vi "Accelerator_DAQ_Small.vi"() -> ()   [LabVIEW 2013]
doc: "Acquire Accelerator Data"
uses:
  <instrlib>/niScope/Controls/niScope vertical coupling.ctl
  <instrlib>/niScope/Controls/niScope trigger slope.ctl
  <instrlib>/niScope/Controls/niScope trigger coupling.ctl
  <instrlib>/niScope/Controls/niScope trigger source.ctl
  Accelerator Measurement/Array_Defctl.ctl
  <vilib>/Utility/error.llb/DialogType.ctl
  <vilib>/Utility/miscctls.llb/LVPointTypeDef.ctl
  Public API/Dust_Event.ctl
  Public API/Signal.ctl
  Private/Role ID.ctl
  Private/Hardware ID.ctl
  Private/Estimate_source.ctl
  Functional Global Variables/Action Items.ctl
  <vilib>/Analysis/baseanly.llb/Mean (DBL).vi
  Private/PSU updated.vi
  <vilib>/addons/database/Connection.llb/Conn Execute.vi
  <vilib>/addons/database/Recordset.llb/Rec Fetch Recordset Data (R).vi
  <vilib>/addons/database/Recordset.llb/Rec Destroy - Connection.vi
  <instrlib>/niScope/Configure/Trigger/niScope Configure Trigger Edge.vi
  <instrlib>/niScope/Acquire/Fetch/niScope Multi Fetch Cluster.vi
  <vilib>/addons/database/_DB Variant To Data/Database Variant To Data.xnode
  <vilib>/Analysis/NI_AALBase.lvlib
  <vilib>/addons/database/NI_Database_API.lvlib
panel:
  out "Big Accelerator?":bool
  out "Array 2":T1=["Dev1", "Dev2"]
  out "error out 5":errorcluster
  in  "Trigger":enum32{"Edge"}(tab)
  in  "Trigger Source Edge 2":T2="2" caption="Source"
  in  "Trigger Source Edge":T2="0" caption="Source"
  in  "Coupling":T3=1 items=["AC"=0, "DC"=1, "HF Reject"=3, "LF Reject"=4, "AC Plus HF Reject"=1001]
  in  "Slope":T4 caption="Trigger Slope"
  in  "Level":dbl=1.0 caption="Trigger Level" step=0.001 format="%.3f"
  in  "Delay":dbl caption="Trigger Delay" format="%.4p"
  in  "Reference Position (%)":dbl=40.0 caption="Ref Position" format="%.1f"
  in  "Bandwidth":dbl=-1.0 format="%.2f"
  in  "Vertical Coupling":T5=1 items=["AC", "DC", "Ground"]
  in  "Probe Attenuation":dbl=1.0 format="%.1f"
  in  "Vertical Offset":dbl format="%.4f"
  in  "Vertical Range":dbl=5.0 caption="Vertical Range (V)" format="%.2f"
  out "Actual Sample Rate":dbl=10000000.0 format="%.0p"
  in  "Min Record Length":i32=100000 caption="Min. Record Length"
  in  "Min Sample Rate":dbl=80000000.0 caption="Min. Sample Rate" step=1000000.0 format="%.2p"
  out "Actual Record Length":i32=100000
  out "Mass":dbl format="%#_3g"
  in  "Write to Database?":bool=TRUE
  in  "Limit":dbl
  in  "Limit Triggers":bool
  out "Acquisition #":i32
  in  "WFM Tag":string="trace"
  in  "Location":string="G:\\default"
  in  "Write Raw File?":bool
  out "Saving Raw File...":path=path "G:/2012_06_13_verify_timestamp_labview/trace00000"
  out "?":cluster{dbl, dbl}(knob)={0.0549, 2.0} scale=10.0..0.01
  in  "Ideal Time (Cursor)":dbl=2.0 step=0.01 format="%_2f"
  out "Time Between Triggers":dbl
  out "Average Frequency":dbl format="%#_4g"
  out "output cluster":T6
  out "error out 3":errorcluster
  out "# elements in queue":i32
  out "Stop condition":bool=TRUE
  out "created path":path=path "G:/default"
  out "Numeric":i32=92364
  out "error out 2":errorcluster
  out "Calibration":dbl=24700000000000.0
  out "Array":T1=["Dev1", "Dev2"]
  in  "Debug Mode\n(Confusing)":bool
  out "Multi Plot 2":cluster{dbl[], dbl[]}(graph) caption="Multi Plot"
  in  "Acceleration Voltage (MV)":dbl=2.0 format="%_2g"
  out "Charge":dbl format="%#_3g"
  out "Velocity (Est.)":dbl format="%#_6f"
  out "Final Detector (CH3)":waveform(dbl)(graph)={"t0"=timestamp(0 s since 1904-01-01), "dt"=1e-07, "Y"=[]}
  out "Charge Detector/PSU gate (CH2)":waveform(dbl)(graph)={"t0"=timestamp(0 s since 1904-01-01), "dt"=1e-07, "Y"=[]}
  out "Velocity Detectors (CH0 & CH1)":waveform(dbl)[](graph)
  in  "stop":bool=TRUE
  out "error out":errorcluster={"status"=FALSE, "code"=0, "source"="No Error"} {"code" format="%.0x"}
  # "File Parameters"
  # "Error Handling"
  # "Accelerator DAQ"
  # "Trigger"
  # "Channel"
  # "Vertical"
  # "Horizontal"
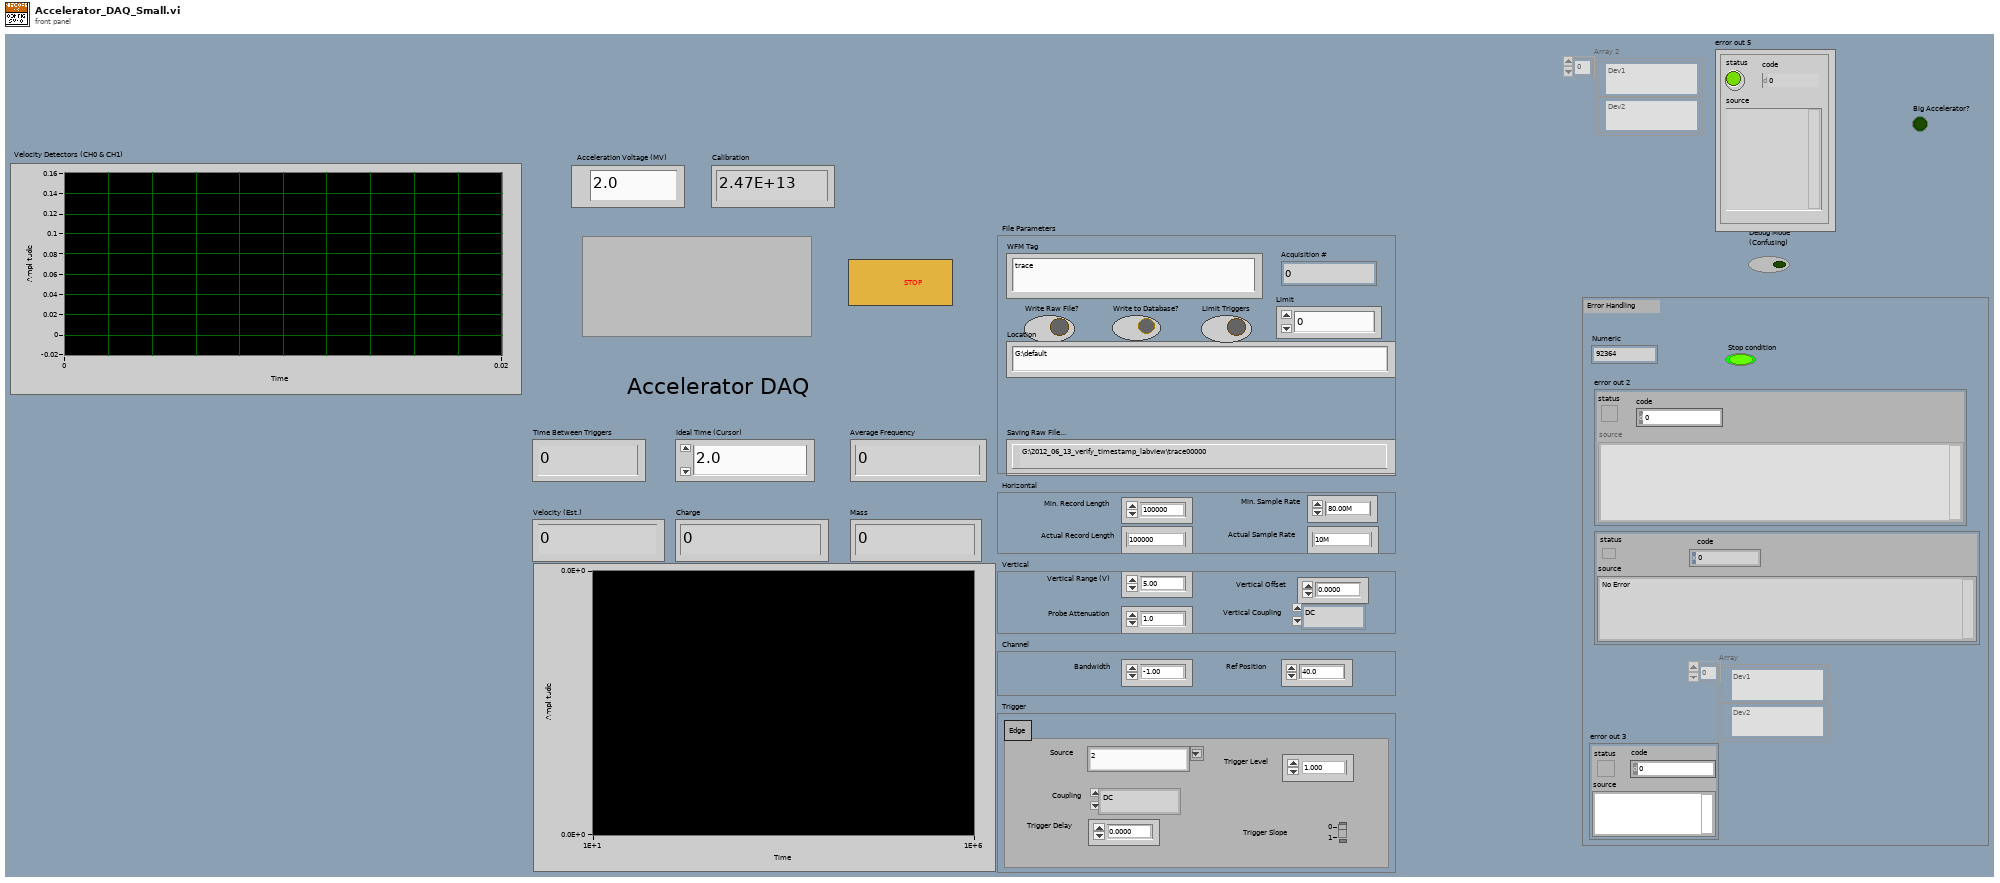
[diagram p1: front panel]
types:
  T1 = typedef "Array_Defctl.ctl" = refnum<k15>[]
  T2 = typedef "niScope trigger source.ctl" = string
  T3 = typedef "niScope trigger coupling.ctl" = u16
  T4 = typedef "niScope trigger slope.ctl" = i32
  T5 = typedef "niScope vertical coupling.ctl" = i32
  T6 = cluster{"File Path Control":path, "Array":waveform(dbl)[]}
  T7 = typedef "LVPointTypeDef.ctl" = cluster{"Horizontal":i16, "Vertical":i16}
  T8 = typedef "DialogType.ctl" = u16
  T9 = typedef "LVAllMonitorsDisplayTypeDef.ctl" = cluster{"Bounds":cluster{"Left":i16, "Top":i16, "Right":i16, "Bottom":i16}, "Depth":i16}[]
  T10 = cluster{"Bounds":cluster{"Left":i16, "Top":i16, "Right":i16, "Bottom":i16}, "Depth":i16}
  T11 = cluster{"Left":i16, "Top":i16, "Right":i16, "Bottom":i16}
  T12 = typedef "NI_Database_API.lvlib/Conn ObjectReference.ctl" = refnum<k1>
  T13 = typedef "NI_Database_API.lvlib/Rec ObjectReference.ctl" = refnum<k1>
  T14 = cluster{"Integer Timestamp":dbl, "Max Velocity":dbl, "Min Velocity":dbl}
  T15 = cluster{"first point time":dbl, "xIncrement":dbl, "Waveforms":dbl[]}[]
  T16 = typedef "Dust_Event.ctl" = cluster{"Time Stamp":timestamp, "Velocity":sgl, "Mass":sgl, "Charge":sgl, "Radius":sgl, "Array":T17[], "Dust Event ID":i64, "Passed_3rd_Detector":bool, "Estimate Source":T20, "Estimate Quality":sgl}
  T17 = typedef "Signal.ctl" = cluster{"Signal ID":i64, "Time Stamp":timestamp, "Dust Event ID":i64, "Role ID":T18, "Data":sgl[], "Signal Length":i32, "dt":sgl, "Offset":dbl, "Hardware ID":T19}
  T18 = typedef "Role ID.ctl" = enum16{"First_Detector", "Second_Detector", "Third_Detector", "LeCroy_CH1", "LeCroy_CH2", "LeCroy_CH3", "LeCroy_CH4", "PSU"}
  T19 = typedef "Hardware ID.ctl" = enum16{"Unknown", "CSA 1", "CSA 2", "CSA 3", "CSA 4", "CSA 5", "CSA 6"}
  T20 = typedef "Estimate_source.ctl" = i8
  T21 = typedef "Action Items.ctl" = enum16{"Initialize", "Get", "Set"}
  T22 = cluster{"relativeInitialX":dbl, "xIncrement":dbl, "wfm":dbl[]}[]
  T23 = cluster{"first point time":dbl, "xIncrement":dbl, "Waveforms":dbl[]}
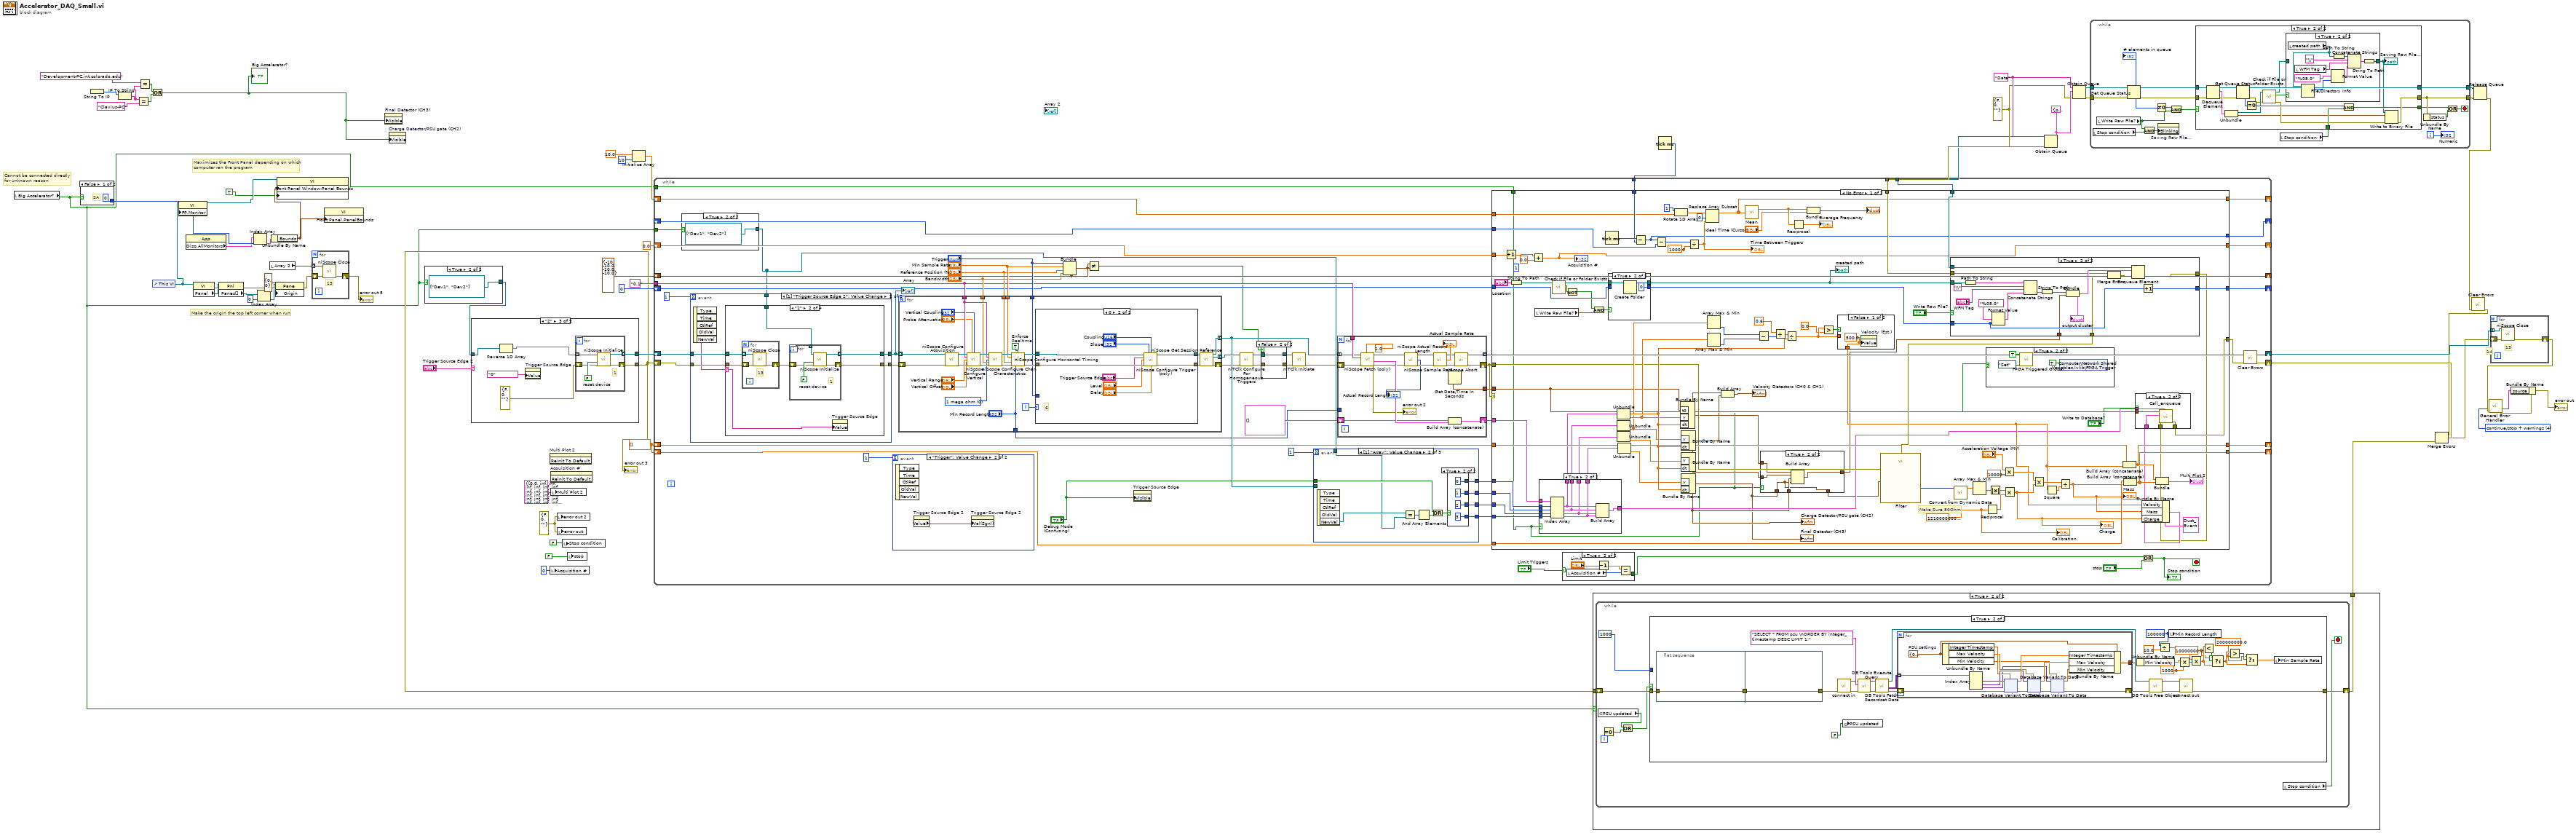
[diagram p0: block diagram]
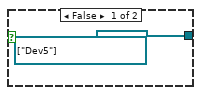
[diagram p2: hidden frame]
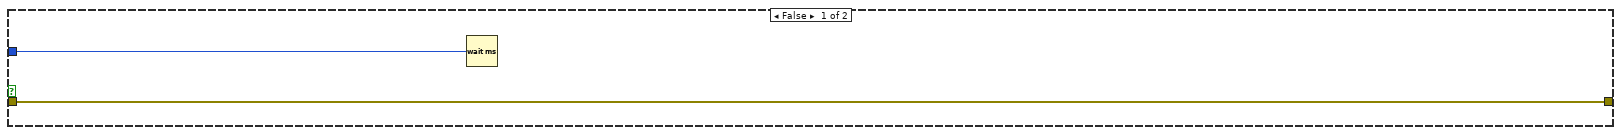
[diagram p4: hidden frame]
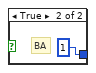
[diagram p5: hidden frame]
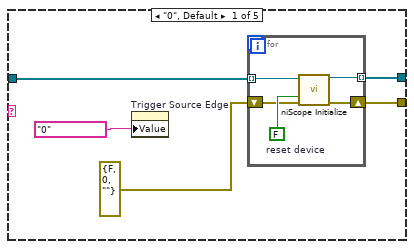
[diagram p6: hidden frame]
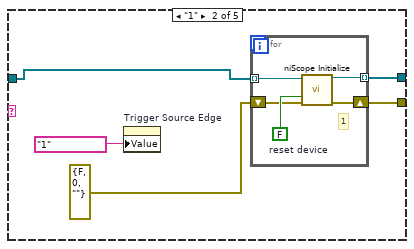
[diagram p7: hidden frame]
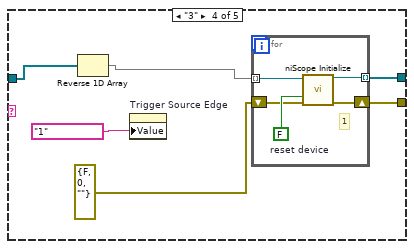
[diagram p8: hidden frame]
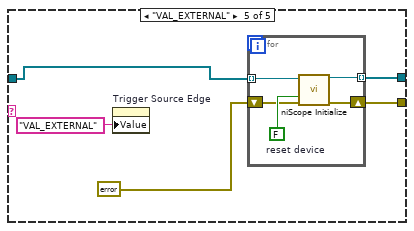
[diagram p9: hidden frame]
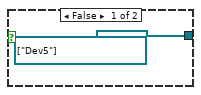
[diagram p10: hidden frame]
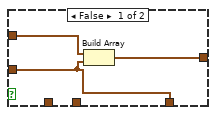
[diagram p11: hidden frame]
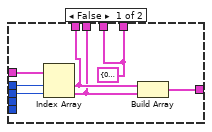
[diagram p12: hidden frame]
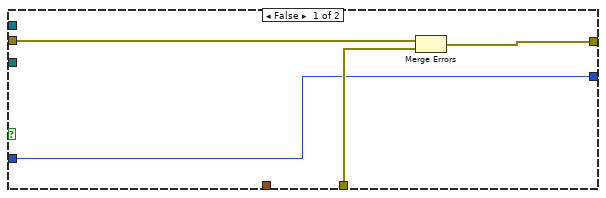
[diagram p16: hidden frame]
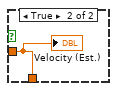
[diagram p17: hidden frame]
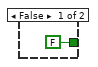
[diagram p19: hidden frame]
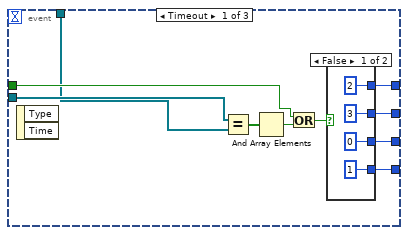
[diagram p20: hidden frame]
diagram:
  w31 = dbl[] []
  w38 = errorcluster {"status"=FALSE, "code"=0, "source"=""} ("error out")
  w42 = errorcluster {"status"=FALSE, "code"=0, "source"=""} ("error out")
  w43 = cluster{path, waveform(sgl)[]} {path "", []} ("output cluster")
  w44 = "Data" ("name (unnamed)")
  w36 = T8 4 items=["no dialog", "OK message", "continue or stop message", "OK message + warnings", "continue/stop + warnings"] ("type of dialog (OK msg:1)")
  # "Cannot be connected directly\nfor unknown reason"
  # "Maximizes the Front Panel depending on which\ncomputer ran the program"
  # "Make the origin the top left corner when run"
  # "14"
  n1 = local read "Big Accelerator?"() -> (w1:bool)
  n2 = case shown="False" w1 {
    tunnel: [0 1] -> w10
    frame False {
      # "SA"
    }
    frame True {
      # "BA"
    }
  }
  n3 = String To IP() -> (0:w16:u32)  [unwired: 1 in]
  n4 = IP To String(2:w16) -> (0:w13:string)  [unwired: 1 in]
  n5 = Equal?(x=w13, y="Clavius-PC") -> (x = y?=w5:bool)
  n6 = Equal?(x="Development-PC.int.colorado.edu", y=w13) -> (x = y?=w4:bool)
  n7 = Or(x=w4, y=w5) -> (x .or. y?=w3:bool)
  "Big Accelerator?" <- w3
  n8 = control-ref of="This VI"() -> (w11:refnum<vi>)
  n9 = property class="VI"(reference=w11, "FP.Monitor"=w10) -> (reference out=w7:refnum<vi>)  [unwired: 1 in, 1 out]
  n10 = property class="App"() -> ("Disp.AllMonitors"=w9:T9)  [unwired: 2 in, 2 out]
  n11 = property class="VI"(reference=w11) -> (error out=w23:errorcluster, "Panel"=w12:refnum<vi>)  [unwired: 1 in, 1 out]
  n12 = property class="Pnl"(reference=w12, error in=w23) -> (error out=w22:errorcluster, "Panes[]"=w21:refnum<vi>[])  [unwired: 1 out]
  n13 = Index Array(array=w9, index=w10) -> (element=w8:T10)
  n14 = Index Array(array=w21, index=0) -> (element=w19:refnum<vi>)
  n15 = local read "Array 2"() -> (w25:T1)
  n16 = Unbundle By Name(w8) -> ("Bounds"=w6:T11)
  n17 = property class="Pane"(reference=w19, error in=w22, "Origin"=T7 {"Horizontal"=0, "Vertical"=0}) -> (error out=w17:errorcluster)  [unwired: 1 out]
  n18 = property class="VI"(reference=w7, "Front Panel Window:Panel Bounds"=w6, "Front Panel Window:Size to Screen (Deprecated)"=TRUE) -> ()  [unwired: 1 in, 2 out]
  n19 = for {
    tunnel: w25 -> [w66] mode=indexing
    shift-right: [w68] -> w24
    shift-left: w17 -> [w67]
    # "13"
    n20 = call <instrlib>:"niScope Close.vi"("instrument handle"=w66, "error in"=w67) -> ("error out"=w68:errorcluster)  [unwired: 13 in]
  }
  "error out 5" <- w24
  n21 = property class="VI"("Front Panel.PanelBounds"=w6) -> ()  [unwired: 2 in, 2 out]
  n22 = property on="Final Detector (CH3)" class="WFGraph (strict)"("Visible"=w3) -> ()  [unwired: 2 in, 2 out]
  n23 = property on="Charge Detector/PSU gate (CH2)" class="WFGraph (strict)"("Visible"=w3) -> ()  [unwired: 2 in, 2 out]
  n24 = case shown="True" w1 {
    tunnel: [refnum<k15>[] ["Dev5"] ("Resources") refnum<k15>[] ["Dev1", "Dev2"] ("Resources")] -> w26
    frame False {
    }
    frame True {
    }
  }
  n25 = case shown="\"2\"" "Trigger Source Edge 2" {
    tunnel: [w75 w84 w95 w106 w117] -> w62
    tunnel: [w74 w83 w94 w105 w116] -> w29
    tunnel: w26 -> [w71 w81 w92 w103 w113]
    frame "0", Default {
      n26 = property on="Trigger Source Edge" class="CmbBox (strict)"("Value"=T2 "0" ("Trigger Source Edge")) -> ()  [unwired: 2 in, 2 out]
      n27 = for {
        tunnel: w71 -> [w79] mode=indexing
        tunnel: [w77] -> w75 mode=indexing
        shift-right: [w76] -> w74
        shift-left: errorcluster {"status"=FALSE, "code"=0, "source"=""} ("error out") -> [w78]
        w80 = FALSE  # reset device
        n28 = call <instrlib>:"niScope Initialize.vi"("resource name"=w79, "reset device"=w80, "error in"=w78) -> ("instrument handle"=w77:refnum<k15>, "error out"=w76:errorcluster)  [unwired: 11 in]
      }
    }
    frame "1" {
      n29 = property on="Trigger Source Edge" class="CmbBox (strict)"("Value"=T2 "1" ("Trigger Source Edge")) -> ()  [unwired: 2 in, 2 out]
      n30 = for {
        tunnel: w81 -> [w89] mode=indexing
        tunnel: [w87] -> w84 mode=indexing
        shift-right: [w86] -> w83
        shift-left: errorcluster {"status"=FALSE, "code"=0, "source"=""} ("error out") -> [w88]
        w90 = FALSE  # reset device
        # "1"
        n31 = call <instrlib>:"niScope Initialize.vi"("resource name"=w89, "reset device"=w90, "error in"=w88) -> ("instrument handle"=w87:refnum<k15>, "error out"=w86:errorcluster)  [unwired: 11 in]
      }
    }
    frame "2" {
      n32 = Reverse 1D Array(array=w92) -> (reversed array=w91:refnum<k15>[])
      n33 = property on="Trigger Source Edge" class="CmbBox (strict)"("Value"=T2 "0" ("Trigger Source Edge")) -> ()  [unwired: 2 in, 2 out]
      n34 = for {
        tunnel: w91 -> [w100] mode=indexing
        tunnel: [w98] -> w95 mode=indexing
        shift-right: [w97] -> w94
        shift-left: errorcluster {"status"=FALSE, "code"=0, "source"=""} ("error out") -> [w99]
        w101 = FALSE  # reset device
        # "1"
        n35 = call <instrlib>:"niScope Initialize.vi"("resource name"=w100, "reset device"=w101, "error in"=w99) -> ("instrument handle"=w98:refnum<k15>, "error out"=w97:errorcluster)  [unwired: 11 in]
      }
    }
    frame "3" {
      n36 = Reverse 1D Array(array=w103) -> (reversed array=w102:refnum<k15>[])
      n37 = property on="Trigger Source Edge" class="CmbBox (strict)"("Value"=T2 "1" ("Trigger Source Edge")) -> ()  [unwired: 2 in, 2 out]
      n38 = for {
        tunnel: w102 -> [w111] mode=indexing
        tunnel: [w109] -> w106 mode=indexing
        shift-right: [w108] -> w105
        shift-left: errorcluster {"status"=FALSE, "code"=0, "source"=""} ("error out") -> [w110]
        w112 = FALSE  # reset device
        # "1"
        n39 = call <instrlib>:"niScope Initialize.vi"("resource name"=w111, "reset device"=w112, "error in"=w110) -> ("instrument handle"=w109:refnum<k15>, "error out"=w108:errorcluster)  [unwired: 11 in]
      }
    }
    frame "VAL_EXTERNAL" {
      n40 = property on="Trigger Source Edge" class="CmbBox (strict)"("Value"=T2 "VAL_EXTERNAL" ("Trigger Source Edge")) -> ()  [unwired: 2 in, 2 out]
      n41 = for {
        tunnel: w113 -> [w121] mode=indexing
        tunnel: [w119] -> w117 mode=indexing
        shift-right: [w118] -> w116
        shift-left: errorcluster {"status"=FALSE, "code"=0, "source"=""} ("error out") -> [w120]
        w122 = FALSE  # reset device
        n42 = call <instrlib>:"niScope Initialize.vi"("resource name"=w121, "reset device"=w122, "error in"=w120) -> ("instrument handle"=w119:refnum<k15>, "error out"=w118:errorcluster)  [unwired: 11 in]
      }
    }
  }
  "error out 3" <- w29
  n43 = invoke on="Multi Plot 2" class="XYGraph (strict)" method="Reinit To Default"() -> ()  [unwired: 3 in, 3 out]
  n44 = local write "Acquisition #"(0 ("Acquisition #")) -> ()
  n45 = invoke on="Acquisition #" class="DigNum (strict)" method="Reinit To Default"() -> ()  [unwired: 3 in, 3 out]
  n46 = local write "Multi Plot 2"(cluster{dbl[], dbl[]} {[0.0, inf, inf, inf, inf, inf, inf, inf, inf, inf, inf, inf, inf, inf, inf, inf, inf, inf, inf, inf, inf, inf, inf, inf, inf, inf, inf, inf, inf, inf, inf, inf, inf, inf, inf, inf, inf, inf, inf, inf, inf], [0.0, 0.0, 0.0, 0.0, 0.0, 0.0, 0.0, 0.0, 0.0, 0.0, 0.0, 0.0, 0.0, 0.0, 0.0, 0.0, 0.0, 0.0, 0.0, 0.0, 0.0, 0.0, 0.0, 0.0, 0.0, 0.0, 0.0, 0.0, 0.0, 0.0, 0.0, 0.0, 0.0, 0.0, 0.0, 0.0, 0.0, 0.0, 0.0, 0.0, 0.0]} ("Multi Plot 2")) -> ()
  n47 = local write "error out 2"(w38) -> ()
  n48 = local write "error out"(w38) -> ()
  n49 = local write "Stop condition"(FALSE ("x .or. y?")) -> ()
  n50 = local write "stop"(FALSE ("stop")) -> ()
  n51 = Initialize Array(10.0 ("element"), 10 ("dimension size")) -> (w54:dbl[])
  n52 = case shown="True" w1 {
    tunnel: w29 -> [w123 w125]
    tunnel: [w123 w124] -> w28
    frame False {
    }
    frame True {
      n53 = while {
        shift-right: [w132] -> w124
        shift-left: w125 -> [w133]
        i -> [w131]
        stop <- w130 stop-if-true
        n54 = global read "PSU updated.vi" "PSU updated"() -> (w129:bool)
        n55 = Equal To 0?(x=w131) -> (x = 0?=w127:bool)
        n56 = Or(x=w129, y=w127) -> (x .or. y?=w128:bool)
        n57 = case shown="True" w128 {
          tunnel: w133 -> [w134 w164]
          tunnel: [w134 w163] -> w132
          tunnel: 1000 -> [w135 _]
          frame False {
            n58 = Wait (ms)(milliseconds to wait=w135) -> ()  [unwired: 1 out]
          }
          frame True {
            w137 = 200000000.0 ("y")
            w140 = 10000000.0 ("y")
            w147 = 100000 ("Min Record Length")
            n59 = flat-sequence {
              tunnel: [w166] -> w165
              tunnel: w164 -> [w166]
              tunnel: w165 -> [w167]
              tunnel: [w167] -> w150
              frame #0 {
              }
              frame #1 {
              }
            }
            n60 = call "connect in.vi"("error in (no error)"=w150) -> ("error out"=w154:errorcluster, "Database Connection"=w153:T12)  [unwired: 6 in, 1 out]
            n61 = global write "PSU updated.vi" "PSU updated"(FALSE ("PSU updated")) -> ()
            n62 = call-poly <vilib>:"DB Tools Execute Query.vi"("error in (no error)"=w154, "SQL query"="SELECT * FROM psu \nORDER BY integer_timestamp DESC LIMIT 1;", "connection reference"=w153) -> ("error out"=w156:errorcluster, "recordset reference"=w155:T13)  [unwired: 5 in]
            n63 = call-poly <vilib>:"DB Tools Fetch Recordset Data.vi"("error in (no error)"=w156, "recordset reference"=w155) -> ("error out"=w162:errorcluster, "recordset data"=w161:variant[][], "recordset reference out"=w157:T13)  [unwired: 3 in]
            n64 = for {
              tunnel: w161 -> [w183] mode=indexing
              shift-right: [w168] -> w151
              shift-left: w162 -> [w179]
              tunnel: [w178] -> w152
              w173 = T14 {"Integer Timestamp"=0.0, "Max Velocity"=0.0, "Min Velocity"=0.0}  # PSU settings
              n65 = Unbundle By Name(w173) -> ("Integer Timestamp"=w177:dbl, "Max Velocity"=w174:dbl, "Min Velocity"=w171:dbl)
              n66 = Index Array(array=w183) -> (element #1=w182:variant, element #2=w181:variant, element #3=w172:variant)  [unwired: 3 in]
              n67 = xnode "Database Variant To Data"("database variant"=w182, "error in"=w179, "type"=w177) -> ("data"=w176:dbl, "error out"=w180:errorcluster)
              n68 = xnode "Database Variant To Data"("database variant"=w181, "error in"=w180, "type"=w174) -> ("data"=w175:dbl, "error out"=w169:errorcluster)
              n69 = xnode "Database Variant To Data"("database variant"=w172, "error in"=w169, "type"=w171) -> ("data"=w170:dbl, "error out"=w168:errorcluster)
              n70 = Bundle By Name(cluster=w173, "Integer Timestamp"=w176, "Max Velocity"=w175, "Min Velocity"=w170) -> (w178:T14)
            }
            n71 = Unbundle By Name(w152) -> ("Min Velocity"=w146:dbl)
            n72 = call-poly <vilib>:"DB Tools Free Object.vi"("error in (no error)"=w151, "recordset reference"=w157) -> ("error out"=w158:errorcluster, "connection reference"=w159:T12)  [unwired: 8 in]
            n73 = Divide(x=w147, y=10.0) -> (x/y=w143:dbl)
            n74 = local write "Min Record Length"(w147) -> ()
            n75 = Multiply(x=w146, y=1000.0) -> (x*y=w144:dbl)
            n76 = call "connect out.vi"("error in (no error)"=w158, "connection reference"=w159) -> ("error out"=w163:errorcluster)  [unwired: 9 in]
            n77 = Multiply(x=w143, y=w144) -> (x*y=w141:dbl)
            n78 = Less?(x=w141, y=w140) -> (x < y?=w142:bool)
            n79 = Select(t=w140, s=w142, f=w141) -> (s? t:f=w139:dbl)
            n80 = Greater?(x=w139, y=w137) -> (0:w138:bool)
            n81 = Select(t=w137, s=w138, f=w139) -> (s? t:f=w136:dbl)
            n82 = local write "Min Sample Rate"(w136) -> ()
          }
        }
        n83 = local read "Stop condition"() -> (w130:bool)
      }
    }
  }
  n84 = Tick Count (ms)() -> (millisecond timer value=w57:u32)
  n85 = Obtain Queue(name (unnamed)=w44, element data type=w43, error in (no error)=w42) -> (queue out=w40:refnum<queue>, error out=w51:errorcluster)  [unwired: 2 in, 1 out]
  n86 = while {
    shift-right: [w292] -> w39
    shift-left: w29 -> [w296]
    shift-right: [w330] -> _
    shift-left: cluster{i32, dbl, dbl, dbl} {-10, -10.0, -10.0, -10.0} -> [w331]
    tunnel: w57 -> [w289]
    shift-right: [w287] -> _
    shift-left: w54 -> [w288]
    shift-right: [w286] -> _
    shift-left: _ -> [w290]
    shift-right: [w323] -> _
    shift-left: w31 -> [w300]
    shift-right: [w322] -> _
    shift-left: w31 -> [w321]
    tunnel: "0,1" ("Channel Name") -> [w320]
    shift-right: [w297] -> w52
    shift-left: w62 -> [w318]
    tunnel: w40 -> [w307]
    tunnel: w51 -> [w306]
    shift-right: [w305] -> _
    shift-left: 0 -> [w304]
    shift-right: [w284] -> _
    shift-left: 0.0 -> [w285]
    tunnel: w1 -> [w282]
    tunnel: w1 -> [w280]
    stop <- w295 stop-if-true
    n87 = case shown="True" w280 {
      tunnel: [refnum<k15>[] ["Dev5"] ("Resources") refnum<k15>[] ["Dev1", "Dev2"] ("Resources")] -> w281
      frame False {
      }
      frame True {
      }
    }
    n88 = event shown="[1] \"Trigger Source Edge 2\": Value Change" {
      selector: _ -> [_ _]
      dyn-events: _ -> [_ _]
      timeout: 1 -> [_ _]
      tunnel: w318 -> [w577 w582]
      tunnel: [w577 w580] -> w315
      tunnel: w296 -> [w576 w583]
      tunnel: [w576 w579] -> w316
      tunnel: w281 -> [_ w578]
      event Timeout {
        n89 = event-data() -> ()  [unwired: 1 in, 2 out]
      }
      event Value Change {
        n90 = event-data() -> ("NewVal"=w581:T2)  [unwired: 1 in, 4 out]
        n91 = case shown="\"1\"" w581 {
          selector: w581 -> [w585 w600 _ _]
          tunnel: w582 -> [w587 w602 w620 w634]
          tunnel: [w589 w604 w618 w635] -> w580
          tunnel: w583 -> [w586 w601 w619 w633]
          tunnel: [w588 w603 w617 w636] -> w579
          tunnel: w578 -> [w584 w599 w614 w631]
          frame "0", Default {
            n92 = for {
              tunnel: w587 -> [w591] mode=indexing
              shift-right: [w593] -> w590
              shift-left: w586 -> [w592]
              # "13"
              n93 = call <instrlib>:"niScope Close.vi"("instrument handle"=w591, "error in"=w592) -> ("error out"=w593:errorcluster)  [unwired: 13 in]
            }
            n94 = for {
              tunnel: [w597] -> w589 mode=indexing
              shift-right: [w596] -> w588
              shift-left: w590 -> [w594]
              tunnel: w584 -> [w595] mode=indexing
              w598 = FALSE  # reset device
              # "1"
              n95 = call <instrlib>:"niScope Initialize.vi"("resource name"=w595, "reset device"=w598, "error in"=w594) -> ("instrument handle"=w597:refnum<k15>, "error out"=w596:errorcluster)  [unwired: 11 in]
            }
            n96 = property on="Trigger Source Edge" class="CmbBox (strict)"("Value"=w585) -> ()  [unwired: 2 in, 2 out]
          }
          frame "1" {
            n97 = for {
              tunnel: w602 -> [w606] mode=indexing
              shift-right: [w608] -> w605
              shift-left: w601 -> [w607]
              # "13"
              n98 = call <instrlib>:"niScope Close.vi"("instrument handle"=w606, "error in"=w607) -> ("error out"=w608:errorcluster)  [unwired: 13 in]
            }
            n99 = for {
              tunnel: [w612] -> w604 mode=indexing
              shift-right: [w611] -> w603
              shift-left: w605 -> [w609]
              tunnel: w599 -> [w610] mode=indexing
              w613 = FALSE  # reset device
              # "1"
              n100 = call <instrlib>:"niScope Initialize.vi"("resource name"=w610, "reset device"=w613, "error in"=w609) -> ("instrument handle"=w612:refnum<k15>, "error out"=w611:errorcluster)  [unwired: 11 in]
            }
            n101 = property on="Trigger Source Edge" class="CmbBox (strict)"("Value"=w600) -> ()  [unwired: 2 in, 2 out]
          }
          frame "2" {
            n102 = for {
              tunnel: w620 -> [w622] mode=indexing
              shift-right: [w624] -> w621
              shift-left: w619 -> [w623]
              # "13"
              n103 = call <instrlib>:"niScope Close.vi"("instrument handle"=w622, "error in"=w623) -> ("error out"=w624:errorcluster)  [unwired: 13 in]
            }
            n104 = Reverse 1D Array(array=w614) -> (reversed array=w615:refnum<k15>[])
            n105 = for {
              tunnel: [w628] -> w618 mode=indexing
              shift-right: [w627] -> w617
              shift-left: w621 -> [w625]
              tunnel: w615 -> [w626] mode=indexing
              w629 = FALSE  # reset device
              # "1"
              n106 = call <instrlib>:"niScope Initialize.vi"("resource name"=w626, "reset device"=w629, "error in"=w625) -> ("instrument handle"=w628:refnum<k15>, "error out"=w627:errorcluster)  [unwired: 11 in]
            }
            n107 = property on="Trigger Source Edge" class="CmbBox (strict)"("Value"=T2 "0" ("Trigger Source Edge")) -> ()  [unwired: 2 in, 2 out]
          }
          frame "3" {
            n108 = for {
              tunnel: w634 -> [w638] mode=indexing
              shift-right: [w640] -> w637
              shift-left: w633 -> [w639]
              # "13"
              n109 = call <instrlib>:"niScope Close.vi"("instrument handle"=w638, "error in"=w639) -> ("error out"=w640:errorcluster)  [unwired: 13 in]
            }
            n110 = Reverse 1D Array(array=w631) -> (reversed array=w630:refnum<k15>[])
            n111 = for {
              tunnel: [w644] -> w635 mode=indexing
              shift-right: [w643] -> w636
              shift-left: w637 -> [w641]
              tunnel: w630 -> [w642] mode=indexing
              w645 = FALSE  # reset device
              # "1"
              n112 = call <instrlib>:"niScope Initialize.vi"("resource name"=w642, "reset device"=w645, "error in"=w641) -> ("instrument handle"=w644:refnum<k15>, "error out"=w643:errorcluster)  [unwired: 11 in]
            }
            n113 = property on="Trigger Source Edge" class="CmbBox (strict)"("Value"=T2 "1" ("Trigger Source Edge")) -> ()  [unwired: 2 in, 2 out]
          }
        }
      }
    }
    "Array" <- w315
    n114 = event shown="[1] \"Trigger\": Value Change" {
      selector: _ -> [_ _]
      dyn-events: _ -> [_ _]
      timeout: 1 -> [_ _]
      event Timeout {
        n115 = event-data() -> ()  [unwired: 1 in, 2 out]
      }
      event "Trigger": Value Change {
        n116 = event-data() -> ()  [unwired: 1 in, 5 out]
        n117 = property on="Trigger Source Edge 2" class="CmbBox (strict)"() -> ("Value"=w575:T2)  [unwired: 2 in, 2 out]
        n118 = property on="Trigger Source Edge 2" class="CmbBox (strict)"("Val(Sgnl)"=w575) -> ()  [unwired: 2 in, 2 out]
      }
    }
    n119 = for {
      tunnel: w315 -> [w679] mode=indexing
      shift-right: [w657] -> w327
      shift-left: w316 -> [w678]
      tunnel: w320 -> [w670]
      tunnel: "Min Sample Rate" -> [w663]
      tunnel: "Trigger" -> [w662]
      tunnel: "Bandwidth" -> [w660]
      tunnel: "Reference Position (%)" -> [w659]
      tunnel: [w656] -> w309 mode=indexing
      tunnel: [w655] -> w324 mode=indexing
      tunnel: ["Min Record Length"] -> w308
      i -> [w664]
      w652 = u32 0 items=["1 mega ohm"] ("input impedance")
      w677 = TRUE  # Enforce Realtime
      n120 = call <instrlib>:"niScope Configure Acquisition.vi"("instrument handle"=w679, "error in"=w678) -> ("instrument handle out"=w675:refnum<k15>, "error out"=w676:errorcluster)  [unwired: 12 in]
      n121 = call <instrlib>:"niScope Configure Vertical.vi"("instrument handle"=w675, "probe attenuation"="Probe Attenuation", "vertical coupling"="Vertical Coupling", "channels"=w670, "vertical range"="Vertical Range", "vertical offset"="Vertical Offset", "error in"=w676) -> ("instrument handle out"=w674:refnum<k15>, "error out"=w673:errorcluster)  [unwired: 7 in]
      n122 = call <instrlib>:"niScope Configure Chan Characteristics.vi"("instrument handle"=w674, "channels"=w670, "input impedance"=w652, "maximum input frequency"=w660, "error in"=w673) -> ("instrument handle out"=w671:refnum<k15>, "error out"=w672:errorcluster)  [unwired: 9 in]
      n123 = call <instrlib>:"niScope Configure Horizontal Timing.vi"("instrument handle"=w671, "enforce realtime"=w677, "min sample rate"=w663, "reference position"=w659, "error in"=w672, "min record length"="Min Record Length") -> ("instrument handle out"=w666:refnum<k15>, "error out"=w667:errorcluster)  [unwired: 8 in]
      n124 = case shown="0" w664 {
        tunnel: w667 -> [w680 w690]
        tunnel: w666 -> [w681 w689]
        tunnel: [w681 w688] -> w654
        tunnel: [w680 w687] -> w658
        tunnel: w662 -> [_ _]
        frame 1, Default {
        }
        frame 0 {
          # "6"
          n125 = call-poly <instrlib>:"niScope Configure Trigger (poly).vi"("instrument handle"=w689, "trigger slope"="Slope", "trigger coupling"="Coupling", "trigger source"="Trigger Source Edge", "trigger level"="Level", "error in"=w690, "trigger delay"="Delay") -> ("instrument handle out"=w688:refnum<k15>, "error out"=w687:errorcluster)  [unwired: 7 in]
        }
      }
      n126 = call <instrlib>:"niScope Get Session Reference.vi"("instrument handle"=w654, "error in"=w658) -> ("instrument handle out"=w656:refnum<k15>, "session reference"=w655:refnum<k20>, "error out"=w657:errorcluster)  [unwired: 11 in]
    }
    n127 = Bundle(cluster=w331, "Trigger", "Min Sample Rate", "Reference Position (%)", "Bandwidth") -> (w330:cluster{i32, dbl, dbl, dbl})
    n128 = Not Equal?(x=w331, y=w330) -> (x != y?=w298:bool)
    n129 = property on="Trigger Source Edge" class="CmbBox (strict)"("Visible"="Debug Mode\n(Confusing)") -> ()  [unwired: 2 in, 2 out]
    n130 = call <instrlib>:"niTClk Configure For Homogeneous Triggers.vi"("error in (no error)"=w327, "sessions"=w324) -> ("error out"=w326:errorcluster, "sessions out"=w325:refnum<k20>[])  [unwired: 8 in]
    n131 = case shown="False" w298 {
      tunnel: [w649 w651] -> w336
      tunnel: [w648 w650] -> w335
      tunnel: w325 -> [w646 w651]
      tunnel: w326 -> [w647 w650]
      frame True {
        n132 = call <instrlib>:"niTClk Synchronize.vi"("error in (no error)"=w647, "sessions"=w646) -> ("error out"=w648:errorcluster, "sessions out"=w649:refnum<k20>[])  [unwired: 8 in]
      }
      frame False {
      }
    }
    n133 = call <instrlib>:"niTClk Initiate.vi"("error in (no error)"=w335, "sessions"=w336) -> ("error out"=w337:errorcluster)  [unwired: 8 in, 1 out]
    n134 = event shown="[1] \"Array\": Value Change" {
      selector: _ -> [_ _ _]
      dyn-events: _ -> [_ _ _]
      timeout: 1 -> [_ _ _]
      tunnel: [w533 w550 w566] -> w314
      tunnel: [w532 w549 w565] -> w313
      tunnel: [w531 w548 w564] -> w312
      tunnel: [w530 w547 w563] -> w311
      tunnel: w309 -> [w529 _ _]
      tunnel: "Debug Mode\n(Confusing)" -> [w525 w546 w560]
      tunnel: w281 -> [w524 w542 _]
      event Timeout {
        n135 = event-data() -> ()  [unwired: 1 in, 2 out]
        n136 = Equal?(x=w529, y=w524) -> (x = y?=w528:bool[])
        n137 = And Array Elements(Boolean array=w528) -> (logical AND=w526:bool)
        n138 = Or(x=w525, y=w526) -> (x .or. y?=w527:bool)
        n139 = case shown="False" w527 {
          tunnel: [2 ("index") 0 ("index")] -> w533
          tunnel: [3 ("index") 1 ("index")] -> w532
          tunnel: [0 ("index") 2 ("index")] -> w531
          tunnel: [1 ("index") 3 ("index")] -> w530
          frame False {
          }
          frame True {
          }
        }
      }
      event Value Change {
        n140 = event-data() -> ("NewVal"=w543:T1)  [unwired: 1 in, 4 out]
        n141 = Equal?(x=w543, y=w542) -> (x = y?=w551:bool[])
        n142 = And Array Elements(Boolean array=w551) -> (logical AND=w545:bool)
        n143 = Or(x=w546, y=w545) -> (x .or. y?=w544:bool)
        n144 = case shown="True" w544 {
          tunnel: [2 ("index") 0 ("index")] -> w550
          tunnel: [3 ("index") 1 ("index")] -> w549
          tunnel: [0 ("index") 2 ("index")] -> w548
          tunnel: [1 ("index") 3 ("index")] -> w547
          frame False {
          }
          frame True {
          }
        }
      }
      event "Debug Mode\n(Confusing)": Value Change {
        n145 = event-data() -> ("NewVal"=w561:bool)  [unwired: 1 in, 4 out]
        n146 = Or(x=w561, y=w560) -> (x .or. y?=w562:bool)
        n147 = case shown="True" w562 {
          tunnel: [2 ("index") 0 ("index")] -> w566
          tunnel: [3 ("index") 1 ("index")] -> w565
          tunnel: [0 ("index") 2 ("index")] -> w564
          tunnel: [1 ("index") 3 ("index")] -> w563
          frame False {
          }
          frame True {
          }
        }
      }
    }
    n148 = for {
      tunnel: w320 -> [w519]
      tunnel: w309 -> [w515] mode=indexing
      shift-right: [w523] -> w299
      shift-left: T15 [] ("Waveform Graph") -> [w517]
      shift-right: [w506] -> w283
      shift-left: w337 -> [w516]
      tunnel: w308 -> [_]
      tunnel: [w508] -> w297 mode=indexing
      tunnel: [w514] -> w301
      n149 = call-poly <instrlib>:"niScope Fetch (poly).vi"("timeout"=1.0 ("Timeout (s)"), "error in"=w516, "channels"=w519, "instrument handle"=w515) -> ("error out"=w510:errorcluster, "waveform"=w518:T22, "instrument handle out"=w511:refnum<k15>)  [unwired: 4 in, 1 out]
      "error out 2" <- w510
      n150 = call <instrlib>:"niScope Actual Record Length.vi"("instrument handle"=w511, "error in"=w510) -> ("instrument handle out"=w522:refnum<k15>, "actual record length"=→"Actual Record Length":i32, "error out"=w521:errorcluster)  [unwired: 11 in]
      n151 = call <instrlib>:"niScope Sample Rate.vi"("instrument handle"=w522, "error in"=w521) -> ("instrument handle out"=w509:refnum<k15>, "actual sample rate"=→"Actual Sample Rate":dbl, "error out"=w507:errorcluster)  [unwired: 11 in]
      n152 = Get Date/Time In Seconds() -> (seconds since 1Jan1904=w514:timestamp)
      n153 = Build Array (concatenate)(w517, w518) -> (w523:T22)
      n154 = call <instrlib>:"niScope Abort.vi"("instrument handle"=w509, "error in"=w507) -> ("instrument handle out"=w508:refnum<k15>, "error out"=w506:errorcluster)  [unwired: 12 in]
    }
    n155 = case shown="No Error" w283 {
      tunnel: [w417 w498] -> w323
      tunnel: [w416 w499] -> w322
      tunnel: w321 -> [w415 w499]
      tunnel: w314 -> [w413 _]
      tunnel: w313 -> [w412 _]
      tunnel: w312 -> [w411 _]
      tunnel: w311 -> [w410 _]
      tunnel: w307 -> [w407 _]
      tunnel: w306 -> [w406 _]
      tunnel: [w402 w500] -> w305
      tunnel: w304 -> [w401 w500]
      tunnel: w301 -> [w356 _]
      tunnel: w300 -> [w392 w498]
      tunnel: w299 -> [w383 _]
      tunnel: w283 -> [w378 w497]
      tunnel: [w354 w497] -> w291
      tunnel: w290 -> [w362 w496]
      tunnel: w289 -> [w366 _]
      tunnel: w288 -> [w365 w495]
      tunnel: [w364 w495] -> w287
      tunnel: [w363 w496] -> w286
      tunnel: w285 -> [w359 w494]
      tunnel: [w358 w494] -> w284
      tunnel: w282 -> [w340 _]
      frame No Error {
        w409 = 12100000000000.0 ("x")
        (unwired) 1
        # "Make Sure 50Ohm"
        n156 = Increment(x=w359) -> (x+1=w360:dbl)
        n157 = String To Path(string="Location") -> (path=w404:path)
        n158 = Add(x=w360, y=0.0) -> (x+y=w358:dbl)
        "Acquisition #" <- w358
        n159 = local read "Write Raw File?"() -> (w347:bool)
        n160 = case shown="True" w340 {
          tunnel: w413 -> [w441 w456]
          tunnel: w412 -> [w440 w455]
          tunnel: w411 -> [_ w454]
          tunnel: w410 -> [_ w453]
          tunnel: w383 -> [w445 w452]
          tunnel: [w444 w451] -> w382
          tunnel: [w443 w450] -> w381
          tunnel: [w442 w449] -> w380
          tunnel: [w442 w448] -> w379
          tunnel: [w446 w447] -> w357
          frame False {
            w442 = T23 {"first point time"=0.0, "xIncrement"=0.0, "Waveforms"=[]} ("Waveforms")
            n161 = Index Array(array=w445, index #1=w441, index #2=w440) -> (element #1=w444:T23, element #2=w443:T23)
            n162 = Build Array(w444, w443) -> (w446:T15)
          }
          frame True {
            n163 = Index Array(array=w452, index #1=w456, index #2=w455, index #3=w454, index #4=w453) -> (element #1=w451:T23, element #2=w450:T23, element #3=w449:T23, element #4=w448:T23)
            n164 = Build Array(w451, w450, w449, w448) -> (w447:T15)
          }
        }
        n165 = call <vilib>:"Check if File or Folder Exists.vi"("path"=w404) -> ("file or folder exists?"=w351:bool, "dup path"=w348:path)  [unwired: 8 in, 1 out]
        n166 = Not(x=w351) -> (.not. x?=w350:bool)
        n167 = And(x=w350, y=w347) -> (x .and. y?=w349:bool)
        n168 = Tick Count (ms)() -> (millisecond timer value=w371:u32)
        n169 = case shown="True" w349 {
          tunnel: [w458 w461] -> w393
          tunnel: w348 -> [w458 w460]
          tunnel: w401 -> [w457 _]
          tunnel: [w457 0] -> w400
          frame False {
          }
          frame True {
            n170 = Create Folder(path (use dialog)=w460) -> (created path=w461:path)  [unwired: 2 in, 2 out]
          }
        }
        "created path" <- w393
        n171 = Unbundle(w382) -> ("xIncrement"=w397:dbl, "Waveforms"=w391:dbl[])  [unwired: 1 out]
        n172 = Unbundle(w381) -> ("Waveforms"=w390:dbl[])  [unwired: 2 out]
        n173 = Unbundle(w380) -> ("Waveforms"=w389:dbl[])  [unwired: 2 out]
        n174 = Unbundle(w379) -> ("Waveforms"=w388:dbl[])  [unwired: 2 out]
        n175 = Subtract(x=w371, y=w366) -> (x-y=w363:u32)
        n176 = Subtract(x=w363, y=w362) -> (x-y=w372:u32)
        n177 = Rotate 1D Array(1:w365, 2:1 ("n")) -> (0:w375:dbl[])
        n178 = Bundle By Name("t0"=w356, "Y"=w391, "dt"=w397) -> (w346:waveform(dbl))  [unwired: 1 in]
        n179 = Bundle By Name("Y"=w390, "dt"=w397) -> (w345:waveform(dbl))  [unwired: 1 in]
        n180 = Bundle By Name("Y"=w389, "dt"=w397) -> (w344:waveform(dbl))  [unwired: 1 in]
        "Charge Detector/PSU gate (CH2)" <- w344
        n181 = Bundle By Name("Y"=w388, "dt"=w397) -> (w343:waveform(dbl))  [unwired: 1 in]
        "Final Detector (CH3)" <- w343
        n182 = Divide(x=w372, y=1000.0) -> (x/y=w370:dbl)
        "Time Between Triggers" <- w370
        n183 = Replace Array Subset(array=w375, new element=w370, index=0) -> (w364:dbl[])
        n184 = Array Max & Min(array=w390) -> (min index (indices)=w399:i32)  [unwired: 3 out]
        n185 = Array Max & Min(array=w391) -> (min index (indices)=w398:i32)  [unwired: 3 out]
        n186 = Build Array(w346, w345) -> (→"Velocity Detectors (CH0 & CH1)":waveform(dbl)[])
        n187 = call-poly <vilib>:"Mean.vi"("X"=w364) -> ("mean"=w369:dbl)  [unwired: 1 out]
        n188 = Subtract(x=w399, y=w398) -> (x-y=w430:i32)
        n189 = case shown="True" w340 {
          tunnel: w346 -> [w434 w439]
          tunnel: w345 -> [w433 w438]
          tunnel: w344 -> [_ w437]
          tunnel: w343 -> [_ w436]
          tunnel: [w433 w436] -> w342
          tunnel: [w432 w435] -> w341
          frame False {
            n190 = Build Array(w434, w433) -> (w432:waveform(dbl)[])
          }
          frame True {
            n191 = Build Array(w439, w438, w437, w436) -> (w435:waveform(dbl)[])
          }
        }
        n192 = Divide(x=0.6, y=w430) -> (x/y=w428:dbl)
        n193 = Divide(x=w428, y=w397) -> (x/y=w426:dbl)
        n194 = Reciprocal(x=w369) -> (1/x=→"Average Frequency":dbl)
        n195 = Bundle("mean"=w369, "Ideal Time (Cursor)"="Ideal Time (Cursor)") -> (→"?":cluster{"mean":dbl, "Ideal Time (Cursor)":dbl})  [unwired: 1 in]
        n196 = Greater?(x=w426, y=0.0 ("x")) -> (0:w427:bool)
        n197 = case shown="False" w427 {
          tunnel: w426 -> [_ w493]
          tunnel: [w492 w493] -> w385
          frame False {
            w492 = 500.0 ("Velocity")
            n198 = property on="Velocity (Est.)" class="DigNum (strict)"("Value"=w492) -> ()  [unwired: 2 in, 2 out]
          }
          frame True {
            "Velocity (Est.)" <- w493
          }
        }
        n199 = call "Filter"("error in (no error)"=w378, "Signal"=w342) -> ("error out"=w396:errorcluster, "Filtered Signal"=w414:dynamicdata)  [unwired: 8 in]
        n200 = case shown="True" "Write Raw File?" {
          tunnel: w341 -> [_ w475]
          tunnel: [w472 w489] -> w353
          tunnel: w396 -> [w474 w487]
          tunnel: w407 -> [_ w476]
          tunnel: w406 -> [w473 w485]
          tunnel: w393 -> [_ w483]
          tunnel: [w471 w481] -> w402
          tunnel: w400 -> [w471 w480]
          frame False {
            n201 = Merge Errors(w473, w474) -> (w472:errorcluster)
          }
          frame True {
            n202 = Path To String(path=w483) -> (string=w478:string)
            n203 = Format Value(format string="%05.0", value (0)=w480) -> (output string=w482:string)  [unwired: 1 in]
            n204 = Concatenate Strings(w478, "\\" ("string"), "WFM Tag", w482) -> (w491:string)
            n205 = String To Path(string=w491) -> (path=w484:path)
            n206 = Bundle(w484, w475) -> (w486:cluster{path, waveform(dbl)[]})  [unwired: 1 in]
            "output cluster" <- w486
            n207 = Merge Errors(w485, w487) -> (w488:errorcluster)
            n208 = Enqueue Element(queue=w476, element=w486, error in (no error)=w488) -> (error out=w489:errorcluster)  [unwired: 1 in, 2 out]
            n209 = Increment(x=w480) -> (x+1=w481:i32)
          }
        }
        n210 = call "Convert from Dynamic Data"("Dynamic Data Type"=w414) -> ("Array"=w424:dbl[])  [unwired: 3 in]
        n211 = Array Max & Min(array=w424) -> (min value=w423:dbl)  [unwired: 3 out]
        n212 = Reciprocal(x=w409) -> (1/x=w408:dbl)
        n213 = case shown="True" w340 {
          frame False {
          }
          frame True {
            n214 = call "FPGA Triggered Global.vi"("Action"=Action_Items."Set", "Input"=TRUE) -> ()  [unwired: 9 in, 1 out]
            n215 = shared-variable "My Computer\\Network Shared Variables.lvlib\\FPGA Trigger"(TRUE ("FPGA Trigger")) -> ()  [unwired: 1 in, 1 out]
          }
        }
        n216 = Absolute Value(x=w423) -> (abs(x)=w422:dbl)
        n217 = Multiply(x="Acceleration Voltage (MV)", y=1000000.0) -> (x*y=w394:dbl)
        n218 = Multiply(x=w422, y=w408) -> (x*y=w386:dbl)
        "Charge" <- w386
        n219 = Multiply(x=w394, y=w386) -> (x*y=w421:dbl)
        n220 = Square(x=w385) -> (x^2=w420:dbl)
        n221 = Divide(x=w421, y=w420) -> (x/y=w387:dbl)
        "Mass" <- w387
        n222 = Build Array (concatenate)(w392, w385) -> (w417:dbl[])
        n223 = Build Array (concatenate)(w415, w387) -> (w416:dbl[])
        n224 = Bundle By Name(cluster=T16 {"Time Stamp"=timestamp(0 s since 1904-01-01), "Velocity"=0.0, "Mass"=0.0, "Charge"=0.0, "Radius"=0.0, "Array"=[], "Dust Event ID"=0, "Passed_3rd_Detector"=FALSE, "Estimate Source"=0, "Estimate Quality"=0.0} ("Input Data"), "Velocity"=w385, "Mass"=w387, "Charge"=w386) -> (w355:T16)
        n225 = case shown="True" "Write to Database?" {
          tunnel: w357 -> [_ w470]
          tunnel: w356 -> [_ w469]
          tunnel: w355 -> [_ w468]
          tunnel: [w465 w467] -> w354
          tunnel: w353 -> [w465 w466]
          frame False {
          }
          frame True {
            n226 = call "Call_enqueue.vi"("Waveform"=w470, "error in"=w466, "Input Data"=w468, "seconds since 1Jan1904"=w469) -> ("error IO"=w467:errorcluster)  [unwired: 7 in]
          }
        }
        n227 = Bundle "Bundle"(w417, w416) -> (→"Multi Plot 2":cluster{dbl[], dbl[]})  [unwired: 1 in]
        "Calibration" <- w409
      }
      frame Error {
      }
    }
    n228 = case shown="True" "Limit Triggers" {
      tunnel: [FALSE w504] -> w294
      frame False {
      }
      frame True {
        n229 = local read "Acquisition #"() -> (w503:i32)
        n230 = Decrement(x="Limit") -> (x-1=w502:dbl)
        n231 = Equal?(x=w502, y=w503) -> (x = y?=w504:bool)
      }
    }
    n232 = Or(x=w294, y="stop") -> (x .or. y?=w295:bool)
    "Stop condition" <- w295
    n233 = call <vilib>:"Clear Errors.vi"("error in (no error)"=w291) -> ("error out"=w292:errorcluster)  [unwired: 6 in]
  }
  n234 = Obtain Queue(name (unnamed)=w44, element data type=w43, error in (no error)=w42) -> (queue out=w49:refnum<queue>, error out=w48:errorcluster)  [unwired: 2 in, 1 out]
  n235 = while {
    tunnel: w49 -> [w698]
    tunnel: w48 -> [w691]
    tunnel: [w707] -> w47
    tunnel: [w705] -> w46
    i -> [w701]
    stop <- w704 stop-if-true
    n236 = local read "Stop condition"() -> (w693:bool)
    n237 = local read "Write Raw File?"() -> (w695:bool)
    n238 = Get Queue Status(queue=w698, error in (no error)=w691) -> (queue out=w692:refnum<queue>, error out=w699:errorcluster, # elements in queue=w697:i32)  [unwired: 1 in, 5 out]
    "# elements in queue" <- w697
    n239 = And(x=w695, y=w693) -> (x .and. y?=w706:bool)
    n240 = Not Equal To 0?(x=w697) -> (x != 0?=w696:bool)
    n241 = property on="Saving Raw File..." class="Path"("Blinking"=w706) -> ()  [unwired: 2 in, 2 out]
    n242 = And(x=w696, y=w695) -> (x .and. y?=w700:bool)
    n243 = local read "Stop condition"() -> (w694:bool)
    n244 = case shown="True" w700 {
      tunnel: w692 -> [w711 w730]
      tunnel: [w709 w728] -> w705
      tunnel: [w710 w726] -> w707
      tunnel: w694 -> [w712 w725]
      tunnel: [w712 w722] -> w702
      tunnel: w699 -> [w708 w718]
      frame False {
        n245 = Flush Queue(queue=w711, error in (no error)=w708) -> (queue out=w710:refnum<queue>, error out=w709:errorcluster)  [unwired: 1 out]
      }
      frame True {
        n246 = Dequeue Element(queue=w730, error in (no error)=w718) -> (queue out=w727:refnum<queue>, element=w729:cluster{path, waveform(sgl)[]}, error out=w716:errorcluster)  [unwired: 1 in, 1 out]
        n247 = Unbundle(w729) -> (w717:path, w713:waveform(sgl)[])
        n248 = Get Queue Status(queue=w727, error in (no error)=w716) -> (queue out=w726:refnum<queue>, error out=w715:errorcluster, # elements in queue=w724:i32)  [unwired: 1 in, 5 out]
        n249 = Equal To 0?(x=w724) -> (x = 0?=w723:bool)
        n250 = call <vilib>:"Check if File or Folder Exists.vi"("error in (no error)"=w715, "path"=w717) -> ("error out"=w714:errorcluster, "file or folder exists?"=w721:bool, "dup path"=w720:path)  [unwired: 7 in]
        n251 = case shown="True" w721 {
          tunnel: w720 -> [w731 _]
          tunnel: [w731 w737] -> w719
          frame False {
          }
          frame True {
            n252 = local read "created path"() -> (w734:path)
            n253 = local read "WFM Tag"() -> (w739:string)
            n254 = File/Directory Info(path=w734) -> (size=w735:i64)  [unwired: 1 in, 6 out]
            n255 = Format Value(format string="%05.0", value (0)=w735) -> (output string=w738:string)  [unwired: 1 in]
            n256 = Path To String(path=w734) -> (string=w732:string)
            n257 = Concatenate Strings(w732, "\\" ("string"), w739, w738) -> (w736:string)
            n258 = String To Path(string=w736) -> (path=w737:path)
          }
        }
        "Saving Raw File..." <- w719
        n259 = And(x=w723, y=w725) -> (x .and. y?=w722:bool)
        n260 = Write to Binary File(file (use dialog)=w719, data=w713, error in=w714) -> (error out=w728:errorcluster)  [unwired: 3 in, 2 out]
      }
    }
    n261 = Unbundle By Name(w705) -> ("status"=w703:bool)
    n262 = Or(x=w702, y=w703) -> (x .or. y?=w704:bool)
    "Numeric" <- w701
  }
  n263 = Release Queue(queue=w47, error in (no error)=w46) -> (error out=w34:errorcluster)  [unwired: 1 in, 2 out]
  n264 = call <vilib>:"Clear Errors.vi"("error in (no error)"=w34) -> ("error out"=w33:errorcluster)  [unwired: 6 in]
  n265 = Merge Errors(w33, w39, w28) -> (w35:errorcluster)
  n266 = for {
    tunnel: w52 -> [w741] mode=indexing
    shift-right: [w743] -> w63
    shift-left: w35 -> [w742]
    # "13"
    n267 = call <instrlib>:"niScope Close.vi"("instrument handle"=w741, "error in"=w742) -> ("error out"=w743:errorcluster)  [unwired: 13 in]
  }
  n268 = call <vilib>:"General Error Handler.vi"("type of dialog (OK msg:1)"=w36, "error in (no error)"=w63) -> ("message"=w59:string, "error out"=w61:errorcluster)  [unwired: 9 in, 3 out]
  n269 = Bundle By Name(cluster=w61, "source"=w59) -> (→"error out":errorcluster)
